vi "WriteConf.vi"(2 "error in (no error)":errorcluster, 3 "path":path=path "C:/Users/light/Desktop/ReadParam") -> (0 "error out":errorcluster)   [LabVIEW 2014]
uses:
  <vilib>/Utility/config.llb/Write Key (I32).vi
  <vilib>/Utility/config.llb/NI_LVConfig.lvlib
panel:
  # "1: end"
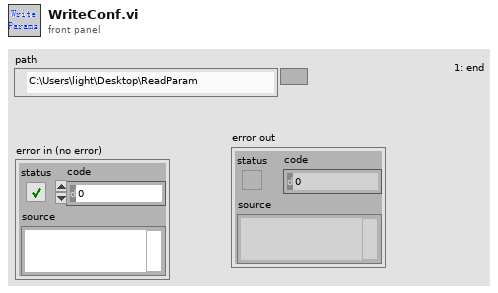
[diagram p1: front panel]
types:
  T1 = typedef "NI_LVConfig.lvlib/Config Data RefNum.ctl" = refnum<k1>
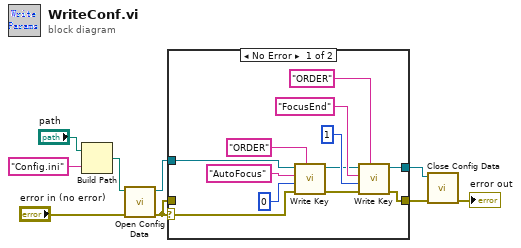
[diagram p0: block diagram]
diagram:
  n1 = Build Path(base path="path", name or relative path="Config.ini") -> (appended path=w3:path)
  n2 = call <vilib>:"Open Config Data.vi"("error in (no error)"="error in (no error)", "configuration file path"=w3) -> ("error out"=w6:errorcluster, "refnum"=w5:T1)  [unwired: 7 in, 1 out]
  n3 = case shown="No Error" w6 {
    selector: w6 -> [w21 _]
    tunnel: [w11 w22] -> w8
    tunnel: [w10 w23] -> w7
    tunnel: w6 -> [_ w23]
    tunnel: w5 -> [w18 w22]
    frame No Error {
      n4 = call-poly <vilib>:"Write Key.vi"("section"="ORDER", "error in (no error)"=w21, "value"=0 ("default value"), "key"="AutoFocus", "refnum"=w18) -> ("error out"=w12:errorcluster, "refnum out"=w13:T1)  [unwired: 4 in, 1 out]
      n5 = call-poly <vilib>:"Write Key.vi"("section"="ORDER", "error in (no error)"=w12, "value"=1 ("default value"), "key"="FocusEnd", "refnum"=w13) -> ("error out"=w10:errorcluster, "refnum out"=w11:T1)  [unwired: 4 in, 1 out]
    }
    frame Error {
    }
  }
  n6 = call <vilib>:"Close Config Data.vi"("error in (no error)"=w7, "refnum"=w8) -> ("error out"=→"error out":errorcluster)  [unwired: 8 in, 1 out]
